vi "PH_Img_BaseClass.set Cam Settings.vi"(0 "i ref in":refnum<vi>, 2 "Cam Settings":T1={"Cam ID"="N/A", "Gain"=nan, "Brightness"=nan, "Shutter"=nan, "Cam Error"=TRUE, "Mode"=-1}, 5 "error in (no error)":errorcluster) -> (14 "i ref out":refnum<vi>, 19 "error out":errorcluster)   [LabVIEW 2014, in "PH_Img_BaseClass.lvlib"]
uses:
  PH_Img_BaseClass.lvlib
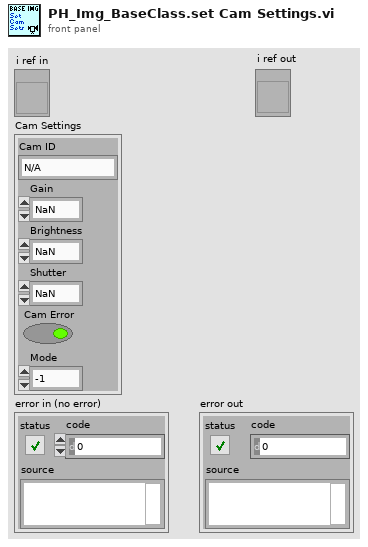
[diagram p1: front panel]
types:
  T1 = cluster{"Cam ID":string, "Gain":dbl, "Brightness":dbl, "Shutter":dbl, "Cam Error":bool, "Mode":i32}
  T2 = typedef "PH_Img_BaseClass.lvlib/PH_Img_BaseClass.i attribute.ctl" = cluster{"GUI Refs":T3, "Timeout Image [ms]":i32, "Default Periodic Period [ms]":i32, "Camera":cluster{"Instancename":string, "Notifier":refnum<notifier>}, "Palette":T4, "Cam Settings":cluster{"Cam ID":string, "Gain":dbl, "Brightness":dbl, "Shutter":dbl, "Cam Info Failure":bool, "Mode":i32}}
  T3 = typedef "PH_Img_BaseClass.lvlib/PH_Img_BaseClass.GUI Refs.ctl" = cluster{"Timeout":refnum<vi>, "Image":refnum<vi>, "Palette":refnum<vi>, "Timeout Set":refnum<vi>}
  T4 = typedef "PH_Img_BaseClass.lvlib/PH_Img_BaseClass.Palette.ctl" = i32
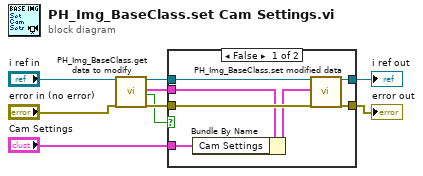
[diagram p0: block diagram]
diagram:
  n1 = call "PH_Img_BaseClass.get data to modify.vi"("i ref in"="i ref in", "error in (no error)"="error in (no error)") -> ("i ref out"=w9:refnum<vi>, "i attribute"=w3:T2, "timed out"=w2:bool, "error out"=w6:errorcluster)  [unwired: 14 in]
  n2 = case shown="False" w2 {
    tunnel: w9 -> [w16 w18]
    tunnel: [w15 w17] -> w7
    tunnel: w6 -> [w14 w17]
    tunnel: [w13 w18] -> w4
    tunnel: w3 -> [w12 _]
    tunnel: "Cam Settings" -> [w10 _]
    frame False {
      n3 = Bundle By Name(cluster=w12, "Cam Settings"=w10) -> (w11:T2)
      n4 = call "PH_Img_BaseClass.set modified data.vi"("i ref in"=w16, "i attribute"=w11, "error in (no error)"=w14) -> ("i ref out"=w13:refnum<vi>, "error out"=w15:errorcluster)  [unwired: 15 in]
    }
    frame True {
    }
  }
  "error out" <- w7
  "i ref out" <- w4
